vi "Client.vi"() -> ()   [LabVIEW 2013]
uses:
  <vilib>/Utility/sysdir.llb/System Directory Type.ctl
panel:
  out "error constant":errorcluster
  out "Array":string[](array[string])
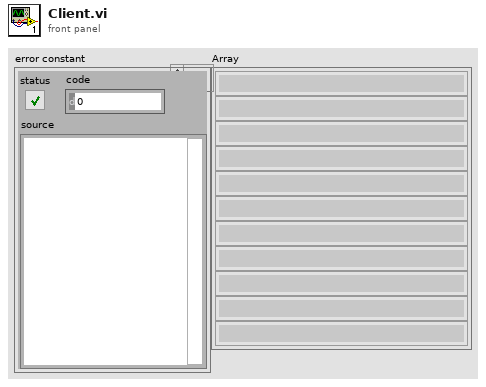
[diagram p1: front panel]
types:
  T1 = enum16{"open", "replace", "create", "open or create", "replace or create", "replace or create with confirmation"}
  T2 = typedef "System Directory Type.ctl" = i32
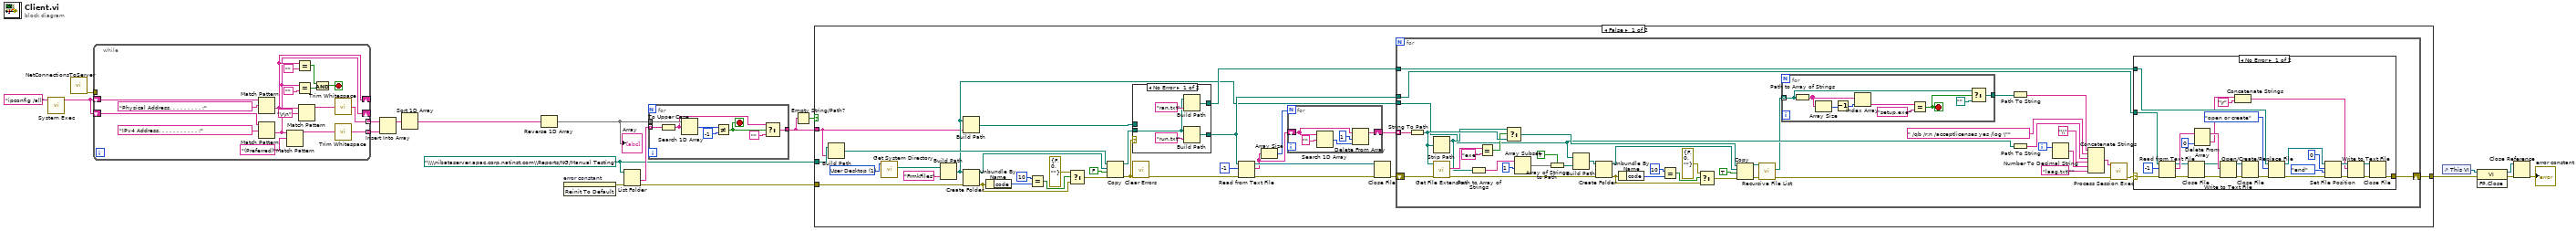
[diagram p0: block diagram]
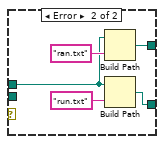
[diagram p2: hidden frame]
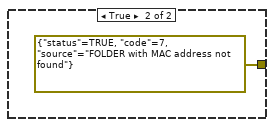
[diagram p4: hidden frame]
diagram:
  w17 = path "\\\\nibataserver.apac.corp.natinst.com\\Reports/NG/Manual Testing" ("path")
  n1 = call <vilib>:"System Exec.vi"("command line"="ipconfig /all") -> ("standard output"=w11:string)  [unwired: 7 in, 3 out]
  n2 = call "NetConnectionsToServer.vi"() -> ("error out"=w12:errorcluster)  [unwired: 11 in]
  n3 = while {
    tunnel: [w30] -> w10 mode=indexing
    shift-right: [w32] -> _
    shift-left: w11 -> [w34]
    tunnel: w12 -> [_]
    shift-right: [w21] -> _
    shift-left: w11 -> [w27]
    tunnel: [w22] -> w9 mode=indexing
    stop <- w23 stop-if-true
    n4 = Match Pattern(string=w34, regular expression="Physical Address. . . . . . . . . :") -> (after substring=w32:string)  [unwired: 1 in, 3 out]
    n5 = Match Pattern(string=w27, regular expression="IPv4 Address. . . . . . . . . . . :") -> (after substring=w21:string)  [unwired: 1 in, 3 out]
    n6 = Match Pattern(string=w21, regular expression="(Preferred)") -> (before substring=w24:string)  [unwired: 1 in, 3 out]
    n7 = Equal?(x=w32, y="") -> (x = y?=w29:bool)
    n8 = Equal?(x=w21, y="") -> (x = y?=w25:bool)
    n9 = Match Pattern(string=w32, regular expression="\r\n") -> (before substring=w31:string)  [unwired: 1 in, 3 out]
    n10 = And(x=w29, y=w25) -> (x .and. y?=w23:bool)
    n11 = call <vilib>:"Trim Whitespace.vi"("string"=w31) -> ("trimmed string"=w30:string)  [unwired: 1 in]
    n12 = call <vilib>:"Trim Whitespace.vi"("string"=w24) -> ("trimmed string"=w22:string)  [unwired: 1 in]
  }
  n13 = Insert Into Array(array=w10, new element=w9) -> (w7:string[])  [unwired: 1 in]
  n14 = Sort 1D Array(array=w7) -> (sorted array=w8:string[])
  n15 = Reverse 1D Array(array=w8) -> (reversed array=w6:string[])
  "Array" <- w6
  n16 = invoke on="error constant" class="Clust (strict)" method="Reinit To Default"() -> (error out=w15:errorcluster)  [unwired: 3 in, 2 out]
  n17 = List Folder(path=w17, error in=w15) -> (folder names=w19:string[], error out=w14:errorcluster)  [unwired: 2 in, 2 out]
  n18 = for {
    tunnel: w19 -> [w38] mode=indexing
    tunnel: w6 -> [w44]
    tunnel: [w39] -> w16
    stop <- w41 stop-if-true
    n19 = To Upper Case(1:w38) -> (0:w37:string)
    n20 = Search 1D Array(1D array=w44, element=w37) -> (index of element=w43:i32)  [unwired: 1 in]
    n21 = Not Equal?(x=w43, y=-1) -> (x != y?=w41:bool)
    n22 = Select(t=w37, s=w41, f="") -> (s? t:f=w39:string)
  }
  n23 = Empty String/Path?(string/path=w16) -> (empty?=w18:bool)
  n24 = case shown="False" w18 {
    tunnel: [w62 errorcluster {"status"=TRUE, "code"=7, "source"="FOLDER with MAC address not found"} ("error constant")] -> w5
    tunnel: w17 -> [w74 _]
    tunnel: w16 -> [w51 _]
    tunnel: w14 -> [w53 _]
    frame False {
      w72 = T2 1 items=["User Home"=0, "User Desktop"=1, "User Documents"=2, "User Application Data"=3, "User Preferences"=4, "User Temporary"=5, "Public Documents"=6, "Public Application Data"=7, "Public Preferences"=8, "Public Cache"=13, "System Core Libraries"=9, "System Installed Libraries"=10, "Application Files"=11, "Boot Volume Root"=12] ("system directory type")
      n25 = Build Path(base path=w74, name or relative path=w51) -> (appended path=w73:path)
      n26 = call <vilib>:"Get System Directory.vi"("system directory type"=w72) -> ("system directory"=w71:path)  [unwired: 10 in]
      n27 = Build Path(base path=w71, name or relative path="FrmkFiles") -> (appended path=w52:path)
      n28 = Build Path(base path=w52, name or relative path=w51) -> (appended path=w50:path)
      n29 = Create Folder(path (use dialog)=w52, error in=w53) -> (created path=w55:path, error out=w68:errorcluster)  [unwired: 1 in, 1 out]
      n30 = Unbundle By Name(w68) -> ("code"=w67:i32)
      n31 = Equal?(x=10, y=w67) -> (x = y?=w65:bool)
      n32 = Select(t=errorcluster {"status"=FALSE, "code"=0, "source"=""} ("error constant"), s=w65, f=w68) -> (s? t:f=w63:errorcluster)
      n33 = Copy(8:w63, 9:FALSE ("overwrite (F)"), 10:w55, 11:w73) -> (0:w49:errorcluster, 3:w54:path)  [unwired: 1 in, 1 out]
      n34 = case shown="No Error" w49 {
        tunnel: [w82 w86] -> w61
        tunnel: [w81 w85] -> w60
        tunnel: w54 -> [w80 _]
        tunnel: w50 -> [_ w87]
        frame No Error {
          n35 = Build Path(base path=w80, name or relative path="ran.txt") -> (appended path=w82:path)
          n36 = Build Path(base path=w80, name or relative path="run.txt") -> (appended path=w81:path)
        }
        frame Error {
          n37 = Build Path(base path=w87, name or relative path="ran.txt") -> (appended path=w86:path)
          n38 = Build Path(base path=w87, name or relative path="run.txt") -> (appended path=w85:path)
        }
      }
      n39 = call <vilib>:"Clear Errors.vi"("error in (no error)"=w49) -> ("error out"=w48:errorcluster)  [unwired: 6 in]
      n40 = Read from Text File(file (use dialog)=w60, count=-1, error in=w48) -> (refnum out=w59:refnum<file>, text=w46:string[], error out=w58:errorcluster)  [unwired: 1 in, 1 out]
      n41 = Array Size(array=w46) -> (size(s)=w47:i32)
      n42 = for {
        N: w47 -> [_]
        shift-right: [w79] -> w45
        shift-left: w46 -> [w78]
        n43 = Search 1D Array(1D array=w78, element="") -> (index of element=w75:i32)  [unwired: 1 in]
        n44 = Delete From Array(array=w78, length=1, index=w75) -> (array with subset deleted=w79:string[])  [unwired: 1 out]
      }
      n45 = Close File(refnum=w59, error in=w58) -> (error out=w57:errorcluster)  [unwired: 1 out]
      n46 = for {
        tunnel: w45 -> [w115] mode=indexing
        tunnel: w52 -> [w107]
        shift-right: [w113] -> w62
        shift-left: w57 -> [w117]
        tunnel: w61 -> [w116]
        tunnel: w60 -> [w114]
        i -> [w95]
        n47 = String To Path(string=w115) -> (path=w128:path)
        n48 = Strip Path(path=w128) -> (stripped path=w111:path)  [unwired: 1 out]
        n49 = call <vilib>:"Get File Extension.vi"("error in (no error)"=w117, "file"=w128) -> ("error out"=w99:errorcluster, "lowercase file extension"=w130:string)  [unwired: 6 in, 2 out]
        n50 = Path to Array of Strings(0:w111) -> (2:w110:string[])  [unwired: 1 out]
        n51 = Equal?(x=w130, y="exe") -> (x = y?=w112:bool)
        n52 = Select(t=w111, s=w112, f=w128) -> (s? t:f=w127:path)
        n53 = Array Subset(array=w110, index=1) -> (w108:string[])  [unwired: 1 in]
        n54 = Array of Strings to Path(0:w108, 1:TRUE ("relative")) -> (2:w106:path)
        n55 = Build Path(base path=w107, name or relative path=w106) -> (appended path=w98:path)
        n56 = Create Folder(path (use dialog)=w98, error in=w99) -> (created path=w97:path, error out=w104:errorcluster)  [unwired: 1 in, 1 out]
        n57 = Unbundle By Name(w104) -> ("code"=w103:i32)
        n58 = Equal?(x=10, y=w103) -> (x = y?=w101:bool)
        n59 = Select(t=errorcluster {"status"=FALSE, "code"=0, "source"=""} ("error constant"), s=w101, f=w104) -> (s? t:f=w96:errorcluster)
        n60 = Copy(8:w96, 9:TRUE ("overwrite (F)"), 10:w97, 11:w127) -> (0:w118:errorcluster, 3:w126:path)  [unwired: 1 in, 1 out]
        n61 = call <vilib>:"Recursive File List.vi"("error in (no error)"=w118, "Folder Path"=w126) -> ("error out"=w119:errorcluster, "All Files in Dir"=w90:path[])  [unwired: 5 in, 3 out]
        n62 = for {
          tunnel: w90 -> [w135] mode=indexing
          tunnel: [w133] -> w124
          stop <- w136 stop-if-true
          n63 = Path to Array of Strings(0:w135) -> (2:w139:string[])  [unwired: 1 out]
          n64 = Array Size(array=w139) -> (size(s)=w131:i32)
          n65 = Decrement(x=w131) -> (x-1=w132:i32)
          n66 = Index Array(array=w139, index=w132) -> (element=w138:string)
          n67 = Equal?(x=w138, y="setup.exe" ("element")) -> (x = y?=w136:bool)
          n68 = Select(t=w135, s=w136, f=path "") -> (s? t:f=w133:path)
        }
        n69 = Path To String(path=w124) -> (string=w125:string)
        n70 = Path To String(path=w107) -> (string=w122:string)
        n71 = Number To Decimal String(number=w95) -> (decimal integer string=w93:string)  [unwired: 1 in]
        n72 = Concatenate Strings(w125, " /qb /r:n /acceptlicenses yes /log \"" ("string"), w122, "\\" ("string"), w93, "laag.txt\"" ("string")) -> (w121:string)
        n73 = call "Process Session Exec.vi"("command line"=w121, "error in (no error)"=w119) -> ("error out"=w120:errorcluster)  [unwired: 9 in, 4 out]
        n74 = case shown="No Error" w120 {
          selector: w120 -> [w140 w167]
          tunnel: w116 -> [w149 _]
          tunnel: w114 -> [w145 _]
          tunnel: [w148 w167] -> w113
          frame No Error {
            n75 = Read from Text File(file (use dialog)=w145, count=-1, error in=w140) -> (refnum out=w146:refnum<file>, text=w165:string[], error out=w147:errorcluster)  [unwired: 1 in, 1 out]
            n76 = Close File(refnum=w146, error in=w147) -> (path=w143:path, error out=w144:errorcluster)
            n77 = Delete From Array(array=w165, index=0) -> (deleted portion=w141:string, array with subset deleted=w164:string[])  [unwired: 1 in]
            n78 = Write to Text File(file (use dialog)=w143, text=w164, error in=w144) -> (refnum out=w153:refnum<file>, error out=w152:errorcluster)  [unwired: 1 in, 1 out]
            n79 = Concatenate Strings(w141, "\r") -> (w156:string)
            n80 = Close File(refnum=w153, error in=w152) -> (error out=w151:errorcluster)  [unwired: 1 out]
            n81 = Open/Create/Replace File(file path (use dialog)=w149, error in=w151, operation (0:open)=T1."open or create") -> (refnum out=w161:refnum<file>, error out=w162:errorcluster)  [unwired: 3 in, 1 out]
            n82 = Set File Position(offset (in bytes) (0)=i64 0, refnum=w161, from (0:start)=enum16{"start", "end", "current"}."end", error in=w162) -> (refnum out=w158:refnum<file>, error out=w157:errorcluster)
            n83 = Write to Text File(file (use dialog)=w158, text=w156, error in=w157) -> (refnum out=w154:refnum<file>, error out=w155:errorcluster)  [unwired: 1 in, 1 out]
            n84 = Close File(refnum=w154, error in=w155) -> (error out=w148:errorcluster)  [unwired: 1 out]
          }
          frame Error {
          }
        }
      }
    }
    frame True {
    }
  }
  n85 = control-ref of="This VI"() -> (w4:refnum<vi>)
  n86 = invoke class="VI" method="FP.Close"(reference=w4, error in=w5) -> (reference out=w3:refnum<vi>, error out=w2:errorcluster)  [unwired: 1 in, 1 out]
  n87 = Close Reference(reference=w3, error in (no error)=w2) -> (error out=→"error constant":errorcluster)
